vi "ep_Broken Rotor Bars Harmonics 1 CH.vi"(0 "spectra":T1, 1 "demodulated? (F)":bool, 2 "search +/- percentage":dbl=0.025, 5 "slip":dbl, 9 "fundamental frequency [Hz]":dbl=50.0, 11 "error in (no error)":errorcluster, 12 "sinc interpolation? (F)":bool, 13 "max sideband order":i32=10) -> (4 "upper sidebands":T2, 6 "lower sidebands":T2, 8 "max sideband magnitude [dB]":dbl, 15 "error out":errorcluster)   [LabVIEW 2014, in "NI_EP_Motor Monitoring.lvlib"]
uses:
  <vilib>/addons/Electrical Power/Motor Monitoring/NI_EP_Motor Monitoring.lvlib
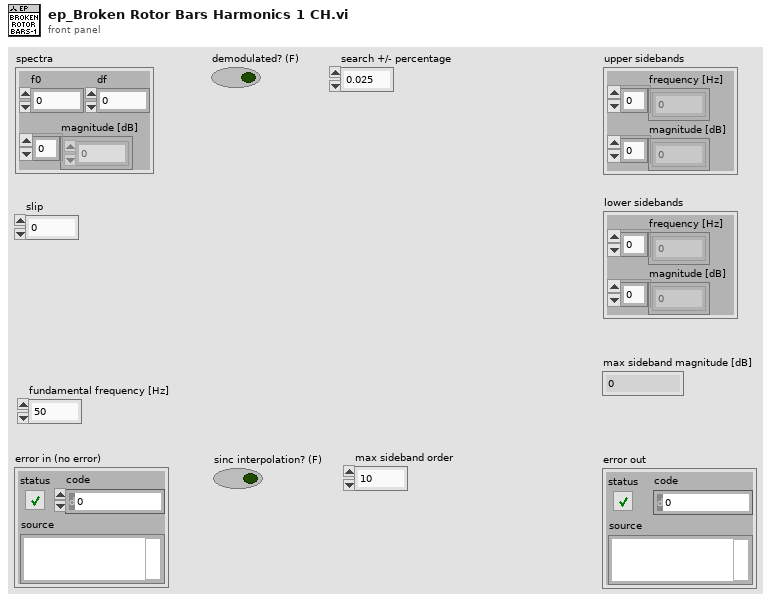
[diagram p1: front panel]
types:
  T1 = cluster{"f0":dbl, "df":dbl, "magnitude [dB]":dbl[]}
  T2 = cluster{"frequency [Hz]":dbl[], "magnitude [dB]":dbl[]}
  T3 = cluster{"min frequency":dbl, "max frequency":dbl, "fs":dbl, "df":dbl, "slip":dbl}
  T4 = cluster{"frequency":dbl[], "magnitude [dB]":dbl[]}
  T5 = cluster{"sideband frequency":dbl, "number of half window length ":u8, "fbrb in range? (F)":bool}
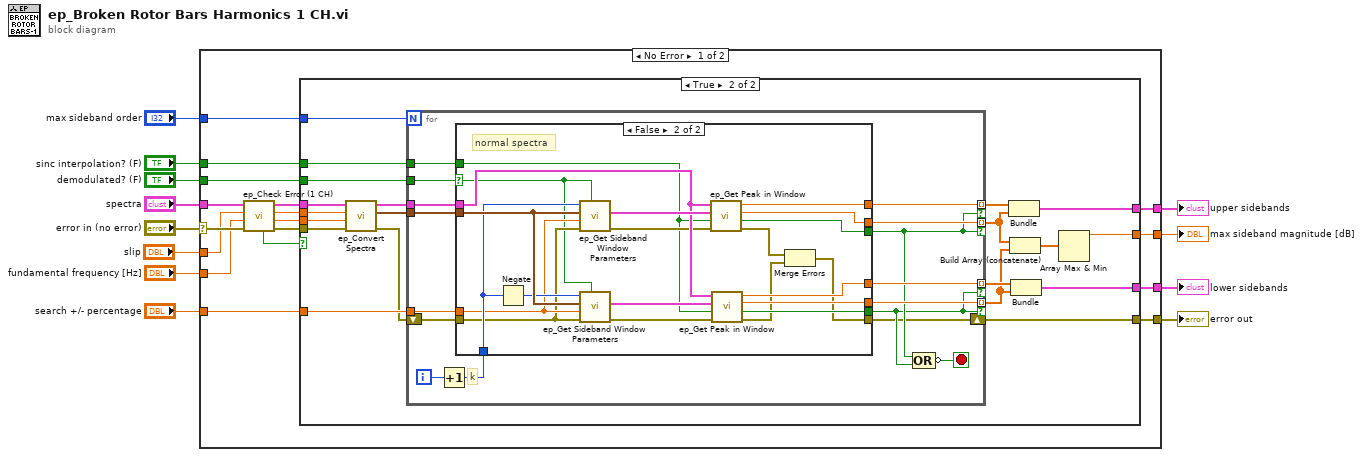
[diagram p0: block diagram]
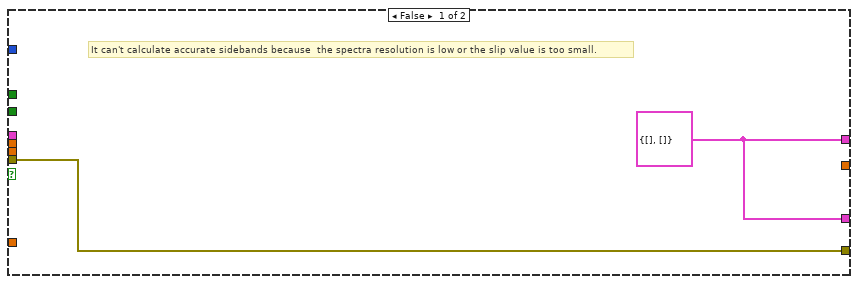
[diagram p2: hidden frame]
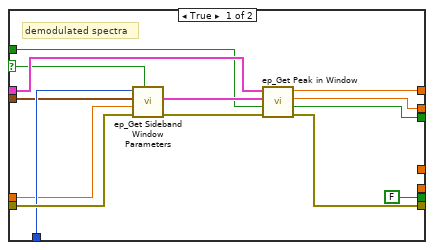
[diagram p3: hidden frame]
diagram:
  n1 = case shown="No Error" "error in (no error)" {
    selector: "error in (no error)" -> [w22 w103]
    tunnel: [w29 _] -> w12
    tunnel: [w28 _] -> w11
    tunnel: "demodulated? (F)" -> [w27 _]
    tunnel: "spectra" -> [w23 _]
    tunnel: "slip" -> [w19 _]
    tunnel: "fundamental frequency [Hz]" -> [w18 _]
    tunnel: [w26 w103] -> w8
    tunnel: "max sideband order" -> [w24 _]
    tunnel: "search +/- percentage" -> [w25 _]
    tunnel: "sinc interpolation? (F)" -> [w17 _]
    tunnel: [w13 _] -> w1
    frame No Error {
      n2 = call <vilib>:"ep_Check Error (1 CH).vi"("error in (no error)"=w22, "fundamental frequency [Hz]"=w18, "slip"=w19, "spectra"=w23) -> ("error out"=w20:errorcluster, "dup fundamental frequency [Hz]"=w14:dbl, "dup slip"=w15:dbl, "dup spectra"=w21:T1, "valid for detection?"=w16:bool)  [unwired: 3 in]
      n3 = case shown="True" w16 {
        tunnel: [w30 w51] -> w29
        tunnel: [w30 w50] -> w28
        tunnel: w27 -> [_ w47]
        tunnel: w21 -> [_ w43]
        tunnel: [w31 w46] -> w26
        tunnel: w25 -> [_ w45]
        tunnel: w24 -> [_ w44]
        tunnel: w20 -> [w31 w41]
        tunnel: w17 -> [_ w38]
        tunnel: w15 -> [_ w37]
        tunnel: w14 -> [_ w36]
        tunnel: [_ w32] -> w13
        frame False {
          w30 = cluster{dbl[], dbl[]} {[], []}
          # "It can't calculate accurate sidebands because  the spectra resolution is low or the slip value is too small."
        }
        frame True {
          n4 = call <vilib>:"ep_Convert Spectra.vi"("error in (no error)"=w41, "fundamental frequency [Hz]"=w36, "slip"=w37, "spectra"=w43) -> ("error out"=w40:errorcluster, "search information"=w39:T3, "spectra points"=w42:T4)  [unwired: 5 in]
          n5 = for {
            N: w44 -> [_]
            tunnel: w42 -> [w67]
            shift-right: [w56] -> w46
            shift-left: w40 -> [w64]
            tunnel: w47 -> [w65]
            tunnel: [w63] -> w48 mode=indexing if=w58
            tunnel: [w62] -> w35 mode=indexing if=w58
            tunnel: [w60] -> w34 mode=indexing if=w57
            tunnel: [w59] -> w49 mode=indexing if=w57
            tunnel: w39 -> [w54]
            tunnel: w45 -> [w53]
            tunnel: w38 -> [w52]
            i -> [w66]
            stop <- w55 stop-if-true
            # "k"
            n6 = Increment(x=w66) -> (x+1=w61:i32)
            n7 = case shown="False" w65 {
              selector: w65 -> [w69 w82]
              tunnel: w67 -> [w81 w94]
              tunnel: [w76 w84] -> w56
              tunnel: w64 -> [w78 w89]
              tunnel: [w80 w102] -> w63
              tunnel: [w79 w101] -> w62
              tunnel: w61 -> [w73 w91]
              tunnel: [w75 w96] -> w58
              tunnel: [_ w100] -> w60
              tunnel: [_ w99] -> w59
              tunnel: [FALSE ("output valid? (F)") w95] -> w57
              tunnel: w54 -> [w71 w93]
              tunnel: w53 -> [w70 w90]
              tunnel: w52 -> [w68 w83]
              frame True {
                # "demodulated spectra"
                n8 = call <vilib>:"ep_Get Sideband Window Parameters.vi"("demodulated? (F)"=w69, "error in (no error)"=w78, "search +/- percentage"=w70, "search information"=w71, "k"=w73) -> ("error out"=w77:errorcluster, "sideband window"=w72:T5)  [unwired: 5 in]
                n9 = call <vilib>:"ep_Get Peak in Window.vi"("error in (no error)"=w77, "sinc interpolation? (F)"=w68, "sideband window"=w72, "spectra points"=w81) -> ("error out"=w76:errorcluster, "output valid? (F)"=w75:bool, "magnitude [dB]"=w79:dbl, "frequency"=w80:dbl)  [unwired: 4 in]
              }
              frame False {
                # "normal spectra"
                n10 = Negate(x=w91) -> (-x=w92:i32)
                n11 = call <vilib>:"ep_Get Sideband Window Parameters.vi"("demodulated? (F)"=w82, "error in (no error)"=w89, "search +/- percentage"=w90, "search information"=w93, "k"=w91) -> ("error out"=w87:errorcluster, "sideband window"=w97:T5)  [unwired: 5 in]
                n12 = call <vilib>:"ep_Get Sideband Window Parameters.vi"("demodulated? (F)"=w82, "error in (no error)"=w89, "search +/- percentage"=w90, "search information"=w93, "k"=w92) -> ("error out"=w88:errorcluster, "sideband window"=w98:T5)  [unwired: 5 in]
                n13 = call <vilib>:"ep_Get Peak in Window.vi"("error in (no error)"=w87, "sinc interpolation? (F)"=w83, "sideband window"=w97, "spectra points"=w94) -> ("error out"=w86:errorcluster, "output valid? (F)"=w96:bool, "magnitude [dB]"=w101:dbl, "frequency"=w102:dbl)  [unwired: 4 in]
                n14 = call <vilib>:"ep_Get Peak in Window.vi"("error in (no error)"=w88, "sinc interpolation? (F)"=w83, "sideband window"=w98, "spectra points"=w94) -> ("error out"=w85:errorcluster, "output valid? (F)"=w95:bool, "magnitude [dB]"=w100:dbl, "frequency"=w99:dbl)  [unwired: 4 in]
                n15 = Merge Errors(w86, w85) -> (w84:errorcluster)
              }
            }
            n16 = Compound Arithmetic op=OR(w58, w57) -> (invert w55:bool)
          }
          n17 = Bundle(w48, w35) -> (w50:cluster{dbl[], dbl[]})  [unwired: 1 in]
          n18 = Build Array (concatenate)(w35, w34) -> (w33:dbl[])
          n19 = Bundle(w49, w34) -> (w51:cluster{dbl[], dbl[]})  [unwired: 1 in]
          n20 = Array Max & Min(array=w33) -> (max value=w32:dbl)  [unwired: 3 out]
        }
      }
    }
    frame Error {
    }
  }
  "lower sidebands" <- w12
  "upper sidebands" <- w11
  "error out" <- w8
  "max sideband magnitude [dB]" <- w1
